vi "Do Request.vi"(7 "Processing In":refnum<class "Processing.lvclass">, 11 "KeepAliveTestController in":refnum<class "KeepAliveTestController.lvclass">) -> (0 "error out":errorcluster, 5 "Processing":refnum<class "Processing.lvclass">)   [LabVIEW 2020, in "Tests.lvlib" / "KeepAliveTestController.lvclass"]
doc: "A controller's main job is to respond to a request by generating a response. The response value must be specified by calling Set Response.vi on the Processing class that's passed through the VI otherwise an error will be generated.\n\nThere are several helpers available for common response types:\nGenerating HTML content programmatically - Create Basic Response.vi\nStreaming a file from disk - Create File Response.vi\nRedirecting the user to another URL - Create Redirect Response.vi\n\nFile responses are streamed in chunks and do not load the entire file into memory at once to send in the response which allows serving large files more efficiently."
uses:
  KeepAliveTestController.lvclass
  HTTP Server/Processing/Processing.lvclass
  HTTP Server/Processing/Processing.lvclass/Processing.ctl
  KeepAliveTestController.lvclass/KeepAliveTestController.ctl
  <vilib>/IlluminatedG/IG HTTP Utils/HTTP Utils/Response/Response.lvclass
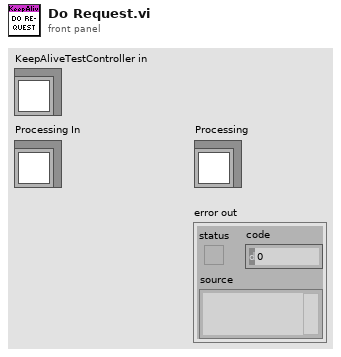
[diagram p1: front panel]
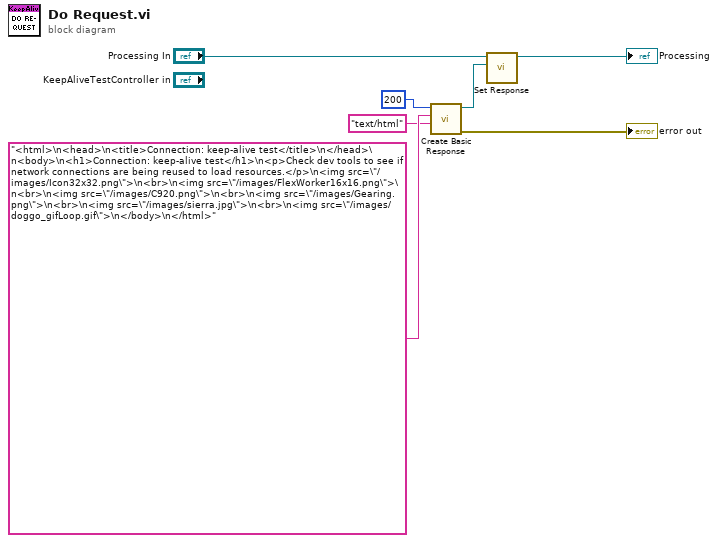
[diagram p0: block diagram]
diagram:
  n1 = call <vilib>:"Create Basic Response.vi"("Content-Type (text/plain)"="text/html", "Payload"="<html>\n<head>\n<title>Connection: keep-alive test</title>\n</head>\n<body>\n<h1>Connection: keep-alive test</h1>\n<p>Check dev tools to see if network connections are being reused to load resources.</p>\n<img src=\"/images/Icon32x32.png\">\n<br>\n<img src=\"/images/FlexWorker16x16.png\">\n<br>\n<img src=\"/images/C920.png\">\n<br>\n<img src=\"/images/Gearing.png\">\n<br>\n<img src=\"/images/sierra.jpg\">\n<br>\n<img src=\"/images/doggo_gifLoop.gif\">\n</body>\n</html>", "Status Code"=u16 200) -> ("error out"=→"error out":errorcluster, "Response out"=w2:refnum<class "Response.lvclass">)  [unwired: 7 in]
  n2 = call "Set Response.vi"("Response"=w2, "Processing in"="Processing In") -> ("Processing out"=→"Processing":refnum<class "Processing.lvclass">)  [unwired: 9 in]
